vi "Dashboard Main.vi"() -> ()   [LabVIEW 2012]
uses:
  <vilib>/event_ctls.llb/eventvkey.ctl
  <vilib>/Utility/miscctls.llb/LVPointTypeDef.ctl
  <vilib>/Utility/config.llb/Read Key (String).vi
  <vilib>/Utility/config.llb/Read Key (I32).vi
  <vilib>/Utility/config.llb/Write Key (String).vi
  <vilib>/Utility/config.llb/Write Key (I32).vi
  <vilib>/Utility/config.llb/NI_LVConfig.lvlib
panel:
  in  "Camera Settings":T1={"Frate Rate"=30, "Compression"=51, "Size"=1} {"Frate Rate" scale=1.0..30.0; "Size" items=["640x480", "320x240", "160x120"]}
  out "Mode":T2(ring)=enum.""
  out "Camera IP":string="0.0.0.11"
  in  "Dashboard Tab":T3(tab)
  out "GO!! GO!! GO!!":bool
  out "Driver Ready":bool
  out "Shooter Speed":T4(ring)
  out "Shooter Encoder\nDead!!":bool
  out "Shooter Good":bool
  out "Dashboard Code Verzion":string
  out "Robot Code Version":string
  out "Display Loop speed (Hz)":dbl
  out "Shooter Good":bool
  out "Shooter Speed":dbl(graph)
  out "Wheel Speed":dbl
  out "Shooter Output":dbl
  out "Shooter Speed":T4(ring)
  out "Left Encoder":dbl
  out "Right Encoder":dbl
  out "Encoder Average":dbl
  out "Left Encoder Rate":dbl
  out "Right Encoder Rate":dbl
  out "Encoder Average Rate":dbl
  out "Gyro":dbl
  out "Battery Value":dbl(slide) scale=0.0..14.0 scale format="%#_2e"
  out "Battery":sgl(graph)
  out "JS1 Z":dbl(slide) scale=-1.0..1.0 scale format="%#_2e"
  out "JS2 Z":dbl(slide) scale=-1.0..1.0 scale format="%#_2e"
  out "Joystick 1":cluster{"X":dbl, "Y":dbl}[](graph)
  out "Joystick 2":cluster{"X":dbl, "Y":dbl}[](graph)
  out "JS Buttons 1":T5
  out "JS Buttons 2":T5
  out "MotorSlide4":dbl(slide) scale=-1.0..1.0 scale format="%#_2e"
  out "MotorSlide3":dbl(slide) scale=-1.0..1.0 scale format="%#_2e"
  out "MotorSlide2":dbl(slide) scale=-1.0..1.0 scale format="%#_2e"
  in  "MotorName3":string="Front Left"
  in  "MotorName4":string="Front Right"
  in  "MotorName1":string="Rear Left"
  in  "MotorName2":string="Rear Right"
  out "MotorChart4":dbl(graph)
  out "MotorChart3":dbl(graph)
  out "MotorChart2":dbl(graph)
  out "MotorSlide1":dbl(slide) scale=-1.0..1.0 scale format="%#_2e"
  out "MotorChart1":dbl(graph)
  out "Robot IP":string="0.0.0.0"
  in  "Slider":dbl(slide) scale=0.0..100.0 scale format="%#_3g"
  in  "On/Off":bool caption="Solenoid"
  in  "Test Name":u16(ring) items=["Select the test to run...", "Example Test", "-------------------------------", "List of tests is built in robot code.", "Replace with your own automated tests."]
  in  "Test Tree":string(tree)
  in  "Motor":cluster{"Value":dbl, "Enable":bool} {"Value" scale=-1.0..1.0 scale format="%#_3g"}
  out "Progress":T6 {"Test Progress" scale=0.0..100.0}
  in  "Rev/Fwd":cluster{"Forward":bool, "Reverse":bool}
  in  "Ring":u16(ring) items=["Auto", "Fixed indoor", "Fixed outdoor 1", "Fixed outdoor 2", "Fixed fluorescent 1", "Fixed fluorescent 2", "Hold current"]
  in  "Debug Mode":bool
  in  "Listbox":i32(listbox)
  in  "Viewer":T7(tab)
  in  "Enable Processing":bool
  out "Mbps":dbl format="%#.1g"
  in  "Enable":bool=TRUE
  in  "DB Camera Config":bool
  out "Mbps":bool
  out "fps":dbl format="%#.1g"
  out "Image Error Message":string="Timeout in Camera Communications"
  out "Camera Image":T8(plugin-control)
  out "Vision Angle":dbl
  out "Buttons 1":cluster{"1":bool, "2":bool, "3":bool}
  out "Kinect 1":cluster{"X":dbl, "Y":dbl, "Z":dbl} {"X" scale=1.0..-1.0; "Y" scale=1.0..-1.0; "Z" scale=1.0..-1.0}
  out "Buttons 2":cluster{"1":bool, "2":bool, "3":bool}
  out "Kinect 2":cluster{"X":dbl, "Y":dbl, "Z":dbl} {"X" scale=1.0..-1.0; "Y" scale=1.0..-1.0; "Z" scale=1.0..-1.0}
  out "Version":string
  out "Skeleton Picture":picture
  out "Players":i8
  out "Tree":string(tree)
  # "Drive & Motors"
  # "Robot IP:"
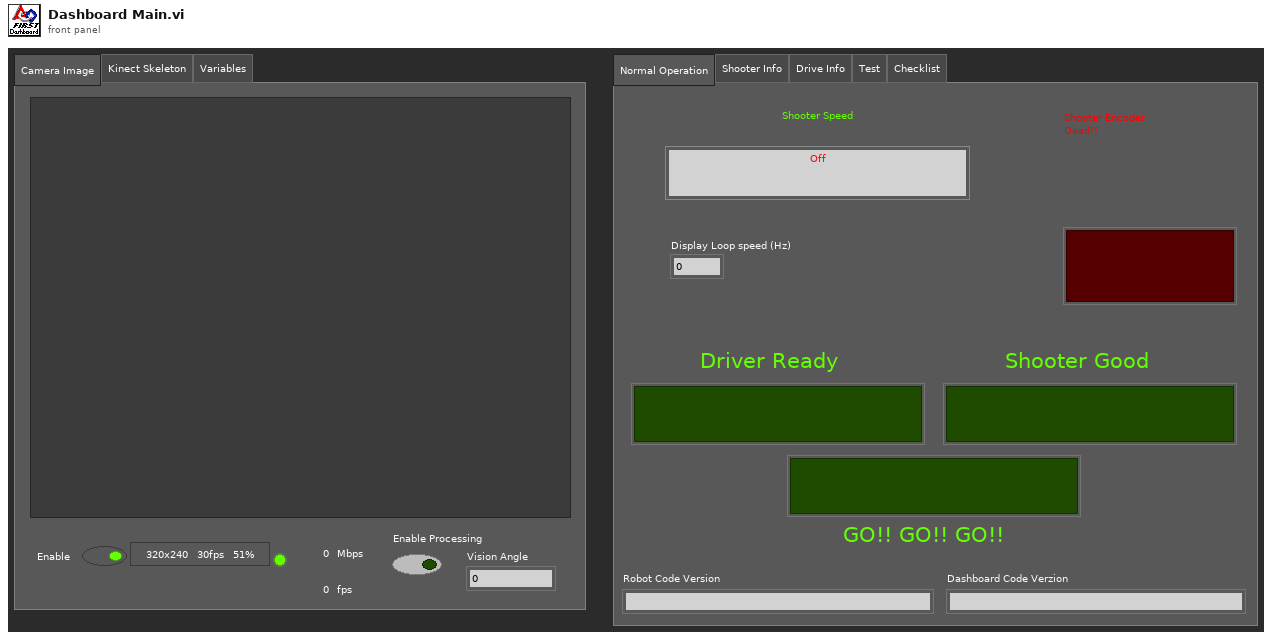
[diagram p1: front panel]
types:
  T1 = cluster{"Frate Rate":i32, "Compression":i32, "Size":u16}
  T2 = enum8{"Tele-Op Disabled", "Tele-Op Enabled", "Auto Disabled", "Auto Enabled", "Test Disabled", "Test Enabled", ""}
  T3 = enum32{"Normal Operation", "Shooter Info", "Drive Info", "Test", "Checklist"}
  T4 = enum16{"Off", "Close Pyramid 3pt", "Far Pyramid 3pt", "Feeder Shot", "UD Far 3pt Shot"}
  T5 = cluster{bool, bool, bool, bool, bool, bool, bool, bool, bool, bool, bool, bool}
  T6 = cluster{"Test Progress":u8, "Test Progress Text":string}
  T7 = enum32{"Camera Image", "Kinect Skeleton", "Variables"}
  T8 = typedef "IMAQ Image.ctl" = refnum<image>
  T9 = typedef "Image Type" = u32
  T10 = cluster{"Competition mode":bool, "Robot Link":bool, "Autonomous":bool, "Enabled":bool, "E-Stop":bool, "Simulated":bool, "TestMode":bool, "Docked Window":bool}
  T11 = cluster{"Boolean Array[0]":bool, "Boolean Array[1]":bool, "Boolean Array[2]":bool, "Boolean Array[3]":bool, "Boolean Array[4]":bool, "Boolean Array[5]":bool, "Boolean Array[6]":bool, "Boolean Array[7]":bool, "Boolean Array[8]":bool, "Boolean Array[9]":bool, "Boolean Array[10]":bool, "Boolean Array[11]":bool}
  T12 = typedef "LVPointTypeDef.ctl" = cluster{"Horizontal":i16, "Vertical":i16}
  T13 = typedef "LVRectTypeDef.ctl" = cluster{"Left":i16, "Top":i16, "Right":i16, "Bottom":i16}
  T14 = typedef "LVBoundsTypeDef.ctl" = cluster{"Width":u32, "Height":u32}
  T15 = typedef "SkeletonTrackState.ctl" = enum32{"NotTracked", "PositionOnly", "Tracked"}
  T16 = cluster{"TrackingState":u8[], "Position":cluster{"x":sgl, "y":sgl, "z":sgl}, cluster{"x":sgl, "y":sgl, "z":sgl, sgl}[], "TrackState":T15}
  T17 = cluster{cluster{"ScaledToPercentRange":dbl, "ScaledToPercentRange":dbl, "ScaledToPercentRange":dbl}, cluster{bool, bool, bool}}[]
  T18 = cluster{cluster{"ScaledToPercentRange":dbl, "ScaledToPercentRange":dbl, "ScaledToPercentRange":dbl}, cluster{bool, bool, bool}}
  T19 = cluster{"ScaledToPercentRange":dbl, "ScaledToPercentRange":dbl, "ScaledToPercentRange":dbl}
  T20 = typedef "NI_LVConfig.lvlib/Config Data RefNum.ctl" = refnum<k1>
  T21 = typedef "eventvkey.ctl" = enum16{"ASCII", "Enter", "Return", "Shift", "Ctrl", "Alt", "Cmd", "Opt", "Caps", "NumLock", "Clear", "Break", "Up", "Down", "Left", "Right", "Insert", "Delete", "Home", "End", "PageUp", "PageDown", "Escape", "Help", "Pause", "ScrollLock", "F1", "F2", "F3", "F4", "F5", "F6", "F7", "F8", "F9", "F10", "F11", "F12", "F13", "F14", "F15", "F16", "F17", "F18", "F19", "F20", "F21", "F22", "F23", "F24", "Play", "VolumeUp", "VolumeDown", "Mute", "Two Byte Char"}
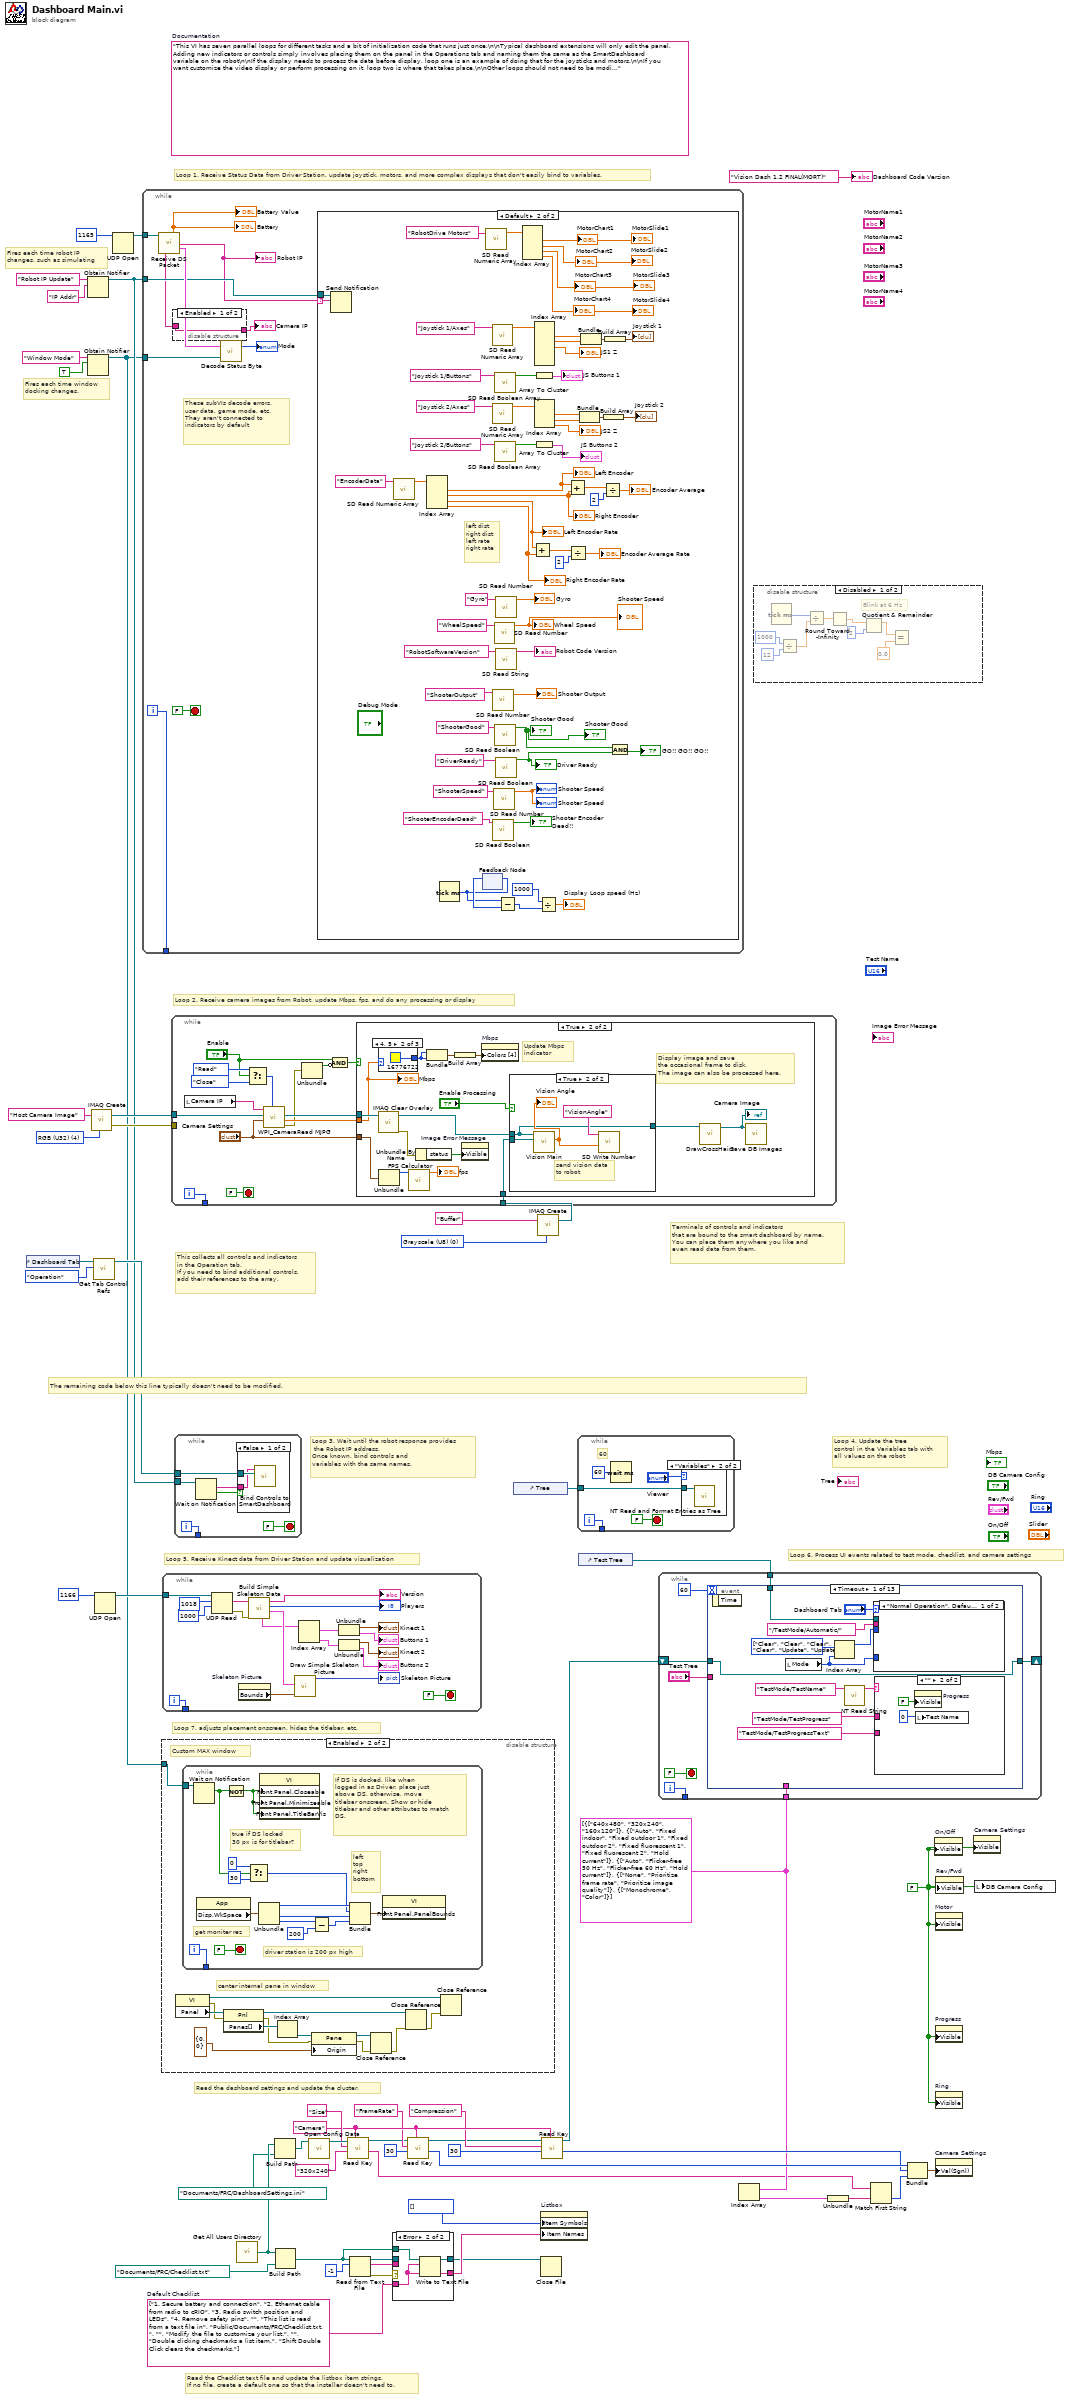
[diagram p0: block diagram]
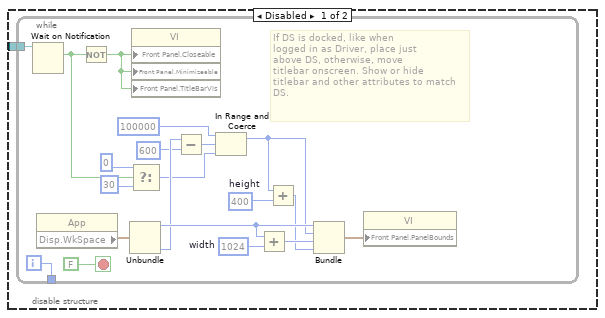
[diagram p3: hidden frame]
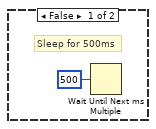
[diagram p5: hidden frame]
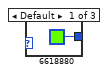
[diagram p7: hidden frame]
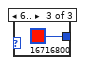
[diagram p8: hidden frame]
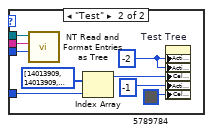
[diagram p10: hidden frame]
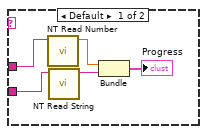
[diagram p11: hidden frame]
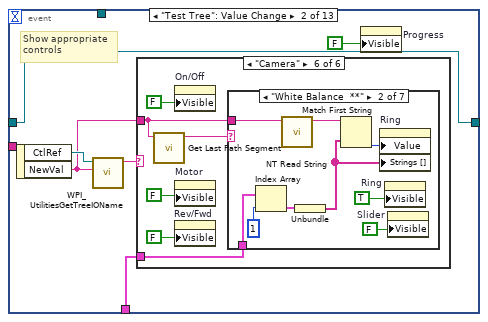
[diagram p12: hidden frame]
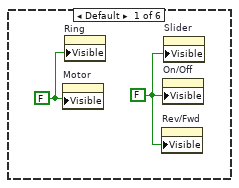
[diagram p13: hidden frame]
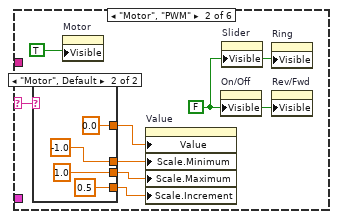
[diagram p14: hidden frame]
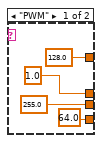
[diagram p15: hidden frame]
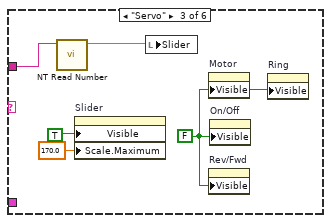
[diagram p16: hidden frame]
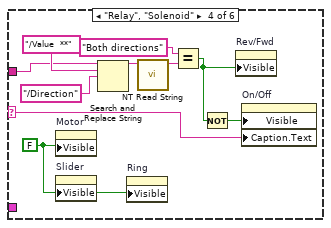
[diagram p17: hidden frame]
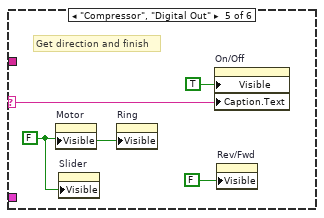
[diagram p18: hidden frame]
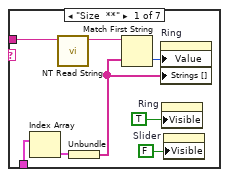
[diagram p19: hidden frame]
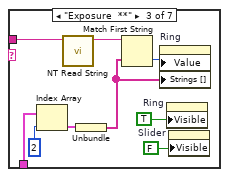
[diagram p20: hidden frame]
diagram:
  w3 = T9 0 items=["Grayscale (U8)", "Grayscale (I16)", "Grayscale (SGL)", "Complex (CSG)", "RGB (U32)", "HSL (U32)", "RGB (U64)", "Grayscale (U16)"] ("Image Type")
  w25 = "Camera"
  w17 = cluster{string[]}[] [{["640x480", "320x240", "160x120"]}, {["Auto", "Fixed indoor", "Fixed outdoor 1", "Fixed outdoor 2", "Fixed fluorescent 1", "Fixed fluorescent 2", "Hold current"]}, {["Auto", "Flicker-free 50 Hz", "Flicker-free 60 Hz", "Hold current"]}, {["None", "Prioritize frame rate", "Prioritize image quality"]}, {["Monochrome", "Color"]}]
  w33 = string[] ["1. Secure battery and connection", "2. Ethernet cable from radio to cRIO", "3. Radio switch position and LEDs", "4. Remove safety pins", "", "This list is read from a text file in", "Public/Documents/FRC/Checklist.txt.", "", "Modify the file to customize your list.", "", "Double clicking checkmarks a list item.", "Shift Double Click clears the checkmarks."]  # Default Checklist
  w31 = FALSE ("Visible")
  (unwired) "This VI has seven parallel loops for different tasks and a bit of initialization code that runs just once.\n\nTypical dashboard extensions will only edit the panel. Adding new indicators or controls simply involves placing them on the panel in the Operations tab and naming them the same as the SmartDashboard variable on the robot\n\nIf the display needs to process the data before display, loop one is an example of doing that for the joysticks and motors.\n\nIf you want customize the video display or perform processing on it, loop two is where that takes place.\n\nOther loops should not need to be modified. They are pretty standard, and document the task they perform."  # Documentation
  w54 = T9 4 items=["Grayscale (U8)", "Grayscale (I16)", "Grayscale (SGL)", "Complex (CSG)", "RGB (U32)", "HSL (U32)", "RGB (U64)"] ("Image Type")
  # "Fires each time robot IP\nchanges, such as simulating"
  # "Fires each time window\ndocking changes."
  # "Read the Checklist text file and update the listbox item strings.\nIf no file, create a default one so that the installer doesn't need to."
  # "This collects all controls and indicators\nin the Operation tab.\nIf you need to bind additional controls,\nadd their references to the array."
  # "The remaining code below this line typically doesn't need to be modified."
  # "Loop 6. Process UI events related to test mode, checklist, and camera settings"
  # "Read the dashboard settings and update the cluster."
  # "Terminals of controls and indicators\nthat are bound to the smart dashboard by name.\nYou can place them anywhere you like and\neven read data from them."
  # "Loop 4. Update the tree\ncontrol in the Variables tab with\nall values on the robot"
  # "Loop 3. Wait until the robot response provides\n the Robot IP address.\nOnce known, bind controls and\nvariables with the same names."
  # "Loop 5. Receive Kinect data from Driver Station and update visualization"
  # "Loop 7. adjusts placement onscreen, hides the titlebar, etc."
  # "Loop 1. Receive Status Data from Driver Station, update joystick, motors, and more complex displays that don't easily bind to variables."
  # "Loop 2. Receive camera images from Robot, update Mbps, fps, and do any processing or display"
  n1 = control-ref of="Dashboard Tab"() -> (w47:refnum<vi>)
  n2 = Obtain Notifier(name (unnamed)="Robot IP Update", notification data type="IP Addr" ("name (unnamed)")) -> (notifier out=w44:refnum<notifier>)  [unwired: 2 in, 2 out]
  n3 = Obtain Notifier(name (unnamed)="Window Mode", notification data type=TRUE) -> (notifier out=w37:refnum<notifier>)  [unwired: 2 in, 2 out]
  n4 = call "IMAQ Create"("Image Name"="Host Camera Image", "Image Type"=w54) -> ("New Image"=w52:T8, "error out"=w51:errorcluster)  [unwired: 2 in, 1 out]
  n5 = call <vilib>:"Get Tab Control Refs.vi"("Page Index"=enum32{"Operation", "Test"}."Operation" ("Dashboard Tab"), "TabControl in"=w47) -> ("ControlsOnPage"=w48:refnum<vi>[])  [unwired: 9 in]
  n6 = UDP Open(11:u16 1166 ("port")) -> (port=w49:refnum<k16>)  [unwired: 2 in, 4 out]
  n7 = UDP Open(11:u16 1165 ("port")) -> (port=w55:refnum<k16>)  [unwired: 2 in, 4 out]
  n8 = while {
    tunnel: w55 -> [w65]
    tunnel: w44 -> [w60]
    tunnel: w37 -> [w63]
    tunnel: [w61] -> _
    i -> [w61]
    stop <- FALSE stop-if-true
    # "These subVIs decode errors, user data, game mode, etc.\nThey aren't connected to indicators by default"
    n9 = call "Receive DS Packet.vi"("Recv Socket"=w65) -> ("Battery"=→"Battery" →"Battery Value":sgl, "Robot IP Address"=w59:string, "Status"=w66:T10, "Camera IP Address"=w57:string)  [unwired: 1 in, 10 out]
    "Robot IP" <- w59
    n10 = disable-structure shown="Enabled" {
      disable-tunnel: [w68 "10.16.76.11" ("Camera IP")] -> w58
      disable-tunnel: w57 -> [w68 _]
      frame Enabled {
      }
      frame Disabled {
      }
    }
    "Camera IP" <- w58
    n11 = call "Decode Status Byte.vi"("Window Mode Notifier"=w63, "Status"=w66) -> ("Mode"=→"Mode":T2)  [unwired: 1 out]
    n12 = case shown="Default" w59 {
      selector: w59 -> [_ w104]
      tunnel: w60 -> [_ w105]
      frame "0.0.0.0" {
        # "Robot not responding, don't poll the variables"
      }
      frame Default {
        # "left dist\nright dist\nleft rate\nright rate"
        n13 = Send Notification(notification=w104, notifier=w105) -> ()  [unwired: 1 in, 2 out]
        n14 = call <vilib>:"SD Read Numeric Array.vi"("Name"="EncoderData") -> ("Numeric Array"=w91:dbl[])  [unwired: 8 in, 2 out]
        n15 = Index Array(array=w91) -> (element #1=w90:dbl, element #2=w89:dbl, element #3=w85:dbl, element #4=w84:dbl)  [unwired: 4 in]
        "Left Encoder" <- w90
        "Right Encoder" <- w89
        "Left Encoder Rate" <- w85
        "Right Encoder Rate" <- w84
        n16 = Tick Count (ms)() -> (millisecond timer value=w73:u32)
        n17 = feedback-in #1(w73) -> ()
        n18 = feedback #1() -> (w74:u32)  [unwired: 1 in]
        n19 = call <vilib>:"SD Read Numeric Array.vi"("Name"="RobotDrive Motors") -> ("Numeric Array"=w128:dbl[])  [unwired: 8 in, 2 out]
        n20 = call <vilib>:"SD Read Numeric Array.vi"("Name"="Joystick 1/Axes") -> ("Numeric Array"=w121:dbl[])  [unwired: 8 in, 2 out]
        n21 = call <vilib>:"SD Read Numeric Array.vi"("Name"="Joystick 2/Axes") -> ("Numeric Array"=w115:dbl[])  [unwired: 8 in, 2 out]
        n22 = call <vilib>:"SD Read Number.vi"("Name"="ShooterOutput") -> ("Numeric"=→"Shooter Output":dbl)  [unwired: 8 in, 2 out]
        n23 = call <vilib>:"SD Read Boolean.vi"("Name"="ShooterEncoderDead") -> ("Boolean"=→"Shooter Encoder\nDead!!":bool)  [unwired: 8 in, 2 out]
        n24 = call <vilib>:"SD Read Number.vi"("Name"="ShooterSpeed") -> ("Numeric"=→"Shooter Speed" →"Shooter Speed":dbl)  [unwired: 8 in, 2 out]
        n25 = call <vilib>:"SD Read Number.vi"("Name"="WheelSpeed") -> ("Numeric"=→"Wheel Speed" →"Shooter Speed":dbl)  [unwired: 8 in, 2 out]
        n26 = call <vilib>:"SD Read Boolean Array.vi"("Name"="Joystick 1/Buttons") -> ("Boolean Array"=w123:bool[])  [unwired: 8 in, 2 out]
        n27 = call <vilib>:"SD Read Boolean Array.vi"("Name"="Joystick 2/Buttons") -> ("Boolean Array"=w114:bool[])  [unwired: 8 in, 2 out]
        n28 = call <vilib>:"SD Read Boolean.vi"("Name"="ShooterGood") -> ("Boolean"=w78:bool)  [unwired: 8 in, 2 out]
        "Shooter Good" <- w78
        "Shooter Good" <- w78
        n29 = call <vilib>:"SD Read Number.vi"("Name"="Gyro") -> ("Numeric"=→"Gyro":dbl)  [unwired: 8 in, 2 out]
        n30 = call <vilib>:"SD Read String.vi"("Name"="RobotSoftwareVersion") -> ("String"=→"Robot Code Version":string)  [unwired: 8 in, 2 out]
        n31 = call <vilib>:"SD Read Boolean.vi"("Name"="DriverReady") -> ("Boolean"=w77:bool)  [unwired: 8 in, 2 out]
        "Driver Ready" <- w77
        n32 = Subtract(x=w73, y=w74) -> (x-y=w72:u32)
        n33 = Index Array(array=w128) -> (element #1=→"MotorChart1" →"MotorSlide1":dbl, element #2=→"MotorSlide2" →"MotorChart2":dbl, element #3=→"MotorChart3" →"MotorSlide3":dbl, element #4=→"MotorChart4" →"MotorSlide4":dbl)  [unwired: 4 in]
        n34 = Add(x=w85, y=w84) -> (x+y=w86:dbl)
        n35 = Array To Cluster(array=w123) -> (cluster=→"JS Buttons 1":T11)
        n36 = Array To Cluster(array=w114) -> (cluster=→"JS Buttons 2":T11)
        n37 = Index Array(array=w121) -> (element #1=w118:dbl, element #2=w119:dbl, element #3=→"JS1 Z":dbl)  [unwired: 6 in, 3 out]
        n38 = Index Array(array=w115) -> (element #1=w110:dbl, element #2=w109:dbl, element #3=→"JS2 Z":dbl)  [unwired: 3 in]
        n39 = Divide(x=1000, y=w72) -> (x/y=→"Display Loop speed (Hz)":dbl)
        n40 = Add(x=w90, y=w89) -> (x+y=w100:dbl)
        n41 = Divide(x=w86, y=2) -> (x/y=→"Encoder Average Rate":dbl)
        n42 = Bundle("Numeric"=w110, "Numeric"=w109) -> (w111:cluster{"Numeric":dbl, "Numeric":dbl})  [unwired: 1 in]
        n43 = Bundle("Numeric"=w118, "Numeric"=w119) -> (w117:cluster{"Numeric":dbl, "Numeric":dbl})  [unwired: 1 in]
        n44 = Divide(x=w100, y=2) -> (x/y=→"Encoder Average":dbl)
        n45 = Build Array(w111) -> (→"Joystick 2":cluster{"Numeric":dbl, "Numeric":dbl}[])
        n46 = Build Array(w117) -> (→"Joystick 1":cluster{"Numeric":dbl, "Numeric":dbl}[])
        n47 = And(x=w78, y=w77) -> (x .and. y?=→"GO!! GO!! GO!!":bool)
      }
    }
  }
  n48 = disable-structure shown="Enabled" {
    disable-tunnel: w37 -> [w132 w165]
    frame Disabled {
      n49 = while {
        tunnel: w132 -> [w151]
        tunnel: [w149] -> _
        i -> [w149]
        stop <- FALSE stop-if-true
        w141 = 1024  # width
        w144 = 400  # height
        # "If DS is docked, like when\nlogged in as Driver, place just\nabove DS, otherwise, move\ntitlebar onscreen. Show or hide\ntitlebar and other attributes to match\nDS."
        n50 = Wait on Notification(notifier=w151) -> (notification=w136:bool)  [unwired: 3 in, 3 out]
        n51 = property class="App"() -> ("Disp.WkSpace"=w147:T13)  [unwired: 2 in, 2 out]
        n52 = Not(x=w136) -> (.not. x?=w150:bool)
        n53 = Unbundle(w147) -> ("Left"=w145:i16, "Bottom"=w142:i16)  [unwired: 2 out]
        n54 = Select(t=0, s=w136, f=30) -> (s? t:f=w135:i32)
        n55 = property class="VI"("Front Panel.Closeable"=w150, "Front Panel.Minimizeable"=w150, "Front Panel.TitleBarVis"=w150) -> ()  [unwired: 2 in, 2 out]
        n56 = Subtract(x=w142, y=600) -> (x-y=w139:i32)
        n57 = In Range and Coerce(upper limit=100000, x=w139, lower limit=w135) -> (coerced(x)=w133:i32)  [unwired: 1 out]
        n58 = Add(x=w145, y=w141) -> (x+y=w146:i32)
        n59 = Add(x=w133, y=w144) -> (x+y=w143:i32)
        n60 = Bundle("Left"=w145, w133, w146, w143) -> (w148:cluster{"Left":i16, i32, i32, i32})  [unwired: 1 out]
        n61 = property class="VI"("Front Panel.PanelBounds"=w148) -> ()  [unwired: 2 in, 2 out]
      }
    }
    frame Enabled {
      # "center internal pane in window"
      # "Custom MAX window"
      n62 = property class="VI"() -> (reference out=w158:refnum<vi>, error out=w157:errorcluster, "Panel"=w164:refnum<vi>)  [unwired: 2 in]
      n63 = while {
        tunnel: w165 -> [w179]
        tunnel: [w177] -> _
        i -> [w177]
        stop <- FALSE stop-if-true
        # "driver station is 200 px high"
        # "true if DS locked\n30 px is for titlebar?"
        # "left\ntop\nright\nbottom"
        # "get moniter rez"
        # "If DS is docked, like when\nlogged in as Driver, place just\nabove DS, otherwise, move\ntitlebar onscreen. Show or hide\ntitlebar and other attributes to match\nDS."
        n64 = Wait on Notification(notifier=w179) -> (notification=w171:bool)  [unwired: 3 in, 3 out]
        n65 = property class="App"() -> ("Disp.WkSpace"=w175:T13)  [unwired: 2 in, 2 out]
        n66 = Not(x=w171) -> (.not. x?=w178:bool)
        n67 = Select(t=0, s=w171, f=30) -> (s? t:f=w169:i32)
        n68 = Unbundle(w175) -> ("Left"=w174:i16, "Right"=w170:i16, "Bottom"=w167:i16)  [unwired: 1 out]
        n69 = property class="VI"("Front Panel.Closeable"=w178, "Front Panel.Minimizeable"=w178, "Front Panel.TitleBarVis"=w178) -> ()  [unwired: 2 in, 2 out]
        n70 = Subtract(x=w167, y=i16 200) -> (x-y=w168:i16)
        n71 = Bundle("Left"=w174, w169, "Right"=w170, w168) -> (w176:cluster{"Left":i16, i32, "Right":i16, i16})  [unwired: 1 out]
        n72 = property class="VI"("Front Panel.PanelBounds"=w176) -> ()  [unwired: 2 in, 2 out]
      }
      n73 = property class="Pnl"(reference=w164, error in=w157) -> (reference out=w159:refnum<vi>, error out=w156:errorcluster, "Panes[]"=w163:refnum<vi>[])
      n74 = Index Array(array=w163) -> (element=w162:refnum<vi>)  [unwired: 1 in]
      n75 = property class="Pane"(reference=w162, error in=w156, "Origin"=T12 {"Horizontal"=0, "Vertical"=0}) -> (reference out=w160:refnum<vi>, error out=w155:errorcluster)
      n76 = Close Reference(reference=w160, error in (no error)=w155) -> (error out=w154:errorcluster)
      n77 = Close Reference(reference=w159, error in (no error)=w154) -> (error out=w153:errorcluster)
      n78 = Close Reference(reference=w158, error in (no error)=w153) -> ()  [unwired: 1 out]
    }
  }
  n79 = while {
    tunnel: w49 -> [w197]
    tunnel: [w182] -> _
    i -> [w182]
    stop <- FALSE stop-if-true
    n80 = UDP Read(connection ID=w197, max size (548)=1018 ("bytes to read"), timeout ms (25000)=1000) -> (data out=w191:string, error out=w181:errorcluster)  [unwired: 1 in, 3 out]
    n81 = property on="Skeleton Picture" class="Pict"() -> ("Bounds"=w193:T14)  [unwired: 2 in, 2 out]
    n82 = call "Build Simple Skeleton Data.vi"("error in (no error)"=w181, "data in"=w191) -> ("Skeleton Data"=w192:T16, "NumPlayers"=→"Players":i8, "Version String"=→"Version":string, "Simple Joystick Info"=w189:T17)  [unwired: 5 in, 1 out]
    n83 = call "Draw Simple Skeleton Picture.vi"("Bounds"=w193, "Simple Skeleton"=w192) -> ("new picture out"=→"Skeleton Picture":picture)  [unwired: 9 in]
    n84 = Index Array(array=w189) -> (element #1=w188:T18, element #2=w187:T18)  [unwired: 2 in]
    n85 = Unbundle(w188) -> (→"Kinect 1":T19, →"Buttons 1":cluster{bool, bool, bool})
    n86 = Unbundle(w187) -> (→"Kinect 2":T19, →"Buttons 2":cluster{bool, bool, bool})
  }
  n87 = while {
    tunnel: w48 -> [w205]
    tunnel: w44 -> [w202]
    tunnel: [w200] -> _
    i -> [w200]
    stop <- FALSE stop-if-true
    n88 = Wait on Notification(notifier=w202) -> (notification=w201:string, timed out?=w203:bool)  [unwired: 3 in, 2 out]
    n89 = case shown="False" w203 {
      tunnel: w205 -> [w207 _]
      tunnel: w201 -> [w206 _]
      frame False {
        n90 = call <vilib>:"Bind Controls to SmartDashboard.vi"("Bound Control Refs"=w207, "Server IP Address"=w206) -> ()  [unwired: 10 in]
      }
      frame True {
      }
    }
  }
  n91 = call "Get All Users Directory.vi"() -> ("All User Path"=w30:path)
  n92 = Build Path(base path=w30, name or relative path=path "Documents/FRC/DashboardSettings.ini") -> (appended path=w29:path)
  n93 = Build Path(base path=w30, name or relative path=path "Documents/FRC/Checklist.txt") -> (appended path=w34:path)
  n94 = call <vilib>:"Open Config Data.vi"("configuration file path"=w29) -> ("refnum"=w28:T20)  [unwired: 8 in, 2 out]
  n95 = call-poly <vilib>:"Read Key.vi"("section"=w25, "default value"="320x240", "key"="Size", "refnum"=w28) -> ("value"=w15:string, "refnum out"=w10:T20)  [unwired: 2 in, 4 out]
  n96 = Read from Text File(file (use dialog)=w34, count=-1 ("timeout ms (25000)")) -> (refnum out=w12:refnum<file>, text=w35:string[], error out=w36:errorcluster)  [unwired: 2 in, 1 out]
  n97 = case shown="Error" w36 {
    tunnel: w35 -> [w209 _]
    tunnel: [w209 w211] -> w32
    tunnel: w33 -> [_ w211]
    tunnel: w34 -> [_ w212]
    tunnel: [w208 w210] -> w11
    tunnel: w12 -> [w208 _]
    frame No Error {
    }
    frame Error {
      n98 = Write to Text File(file (use dialog)=w212, text=w211) -> (refnum out=w210:refnum<file>)  [unwired: 2 in, 2 out]
    }
  }
  n99 = call-poly <vilib>:"Read Key.vi"("section"=w25, "default value"=30, "key"="FrameRate", "refnum"=w10) -> ("value"=w20:i32, "refnum out"=w9:T20)  [unwired: 1 in, 5 out]
  n100 = control-ref of="Tree"() -> (w6:refnum<vi>)
  n101 = call "IMAQ Create"("Image Name"="Buffer", "Image Type"=w3) -> ("New Image"=w2:T8)  [unwired: 3 in, 1 out]
  n102 = while {
    tunnel: w52 -> [w223]
    tunnel: w51 -> [_]
    tunnel: [w226] -> _
    tunnel: w2 -> [w213]
    i -> [w226]
    stop <- FALSE stop-if-true
    n103 = local read "Camera IP"() -> (w225:string)
    n104 = Select(t=enum16{"Read", "Reopen", "Close"}."Read" ("Operation"), s="Enable", f=enum16{"Read", "Reopen", "Close"}."Close" ("Operation")) -> (s? t:f=w218:enum16{"Read", "Reopen", "Close"})
    n105 = call <vilib>:"WPI_CameraRead MJPG.vi"("Operation"=w218, "Camera Settings"="Camera Settings", "Image"=w223, "address"=w225) -> ("error out"=w217:errorcluster, "Bandwidth (kbps)"=w221:dbl, "Image Out"=w222:T8)  [unwired: 5 in]
    n106 = Unbundle(w217) -> ("status"=w215:bool)  [unwired: 2 out]
    n107 = Compound Arithmetic op=AND("Enable", invert w215) -> (w214:bool)
    n108 = case shown="True" w214 {
      tunnel: "Camera Settings" -> [_ w235]
      tunnel: w222 -> [_ w238]
      tunnel: w221 -> [_ w237]
      tunnel: w213 -> [_ w233]
      frame False {
        # "Sleep for 500ms"
        n109 = Wait Until Next ms Multiple(millisecond multiple=u32 500) -> ()  [unwired: 1 out]
      }
      frame True {
        # "Display image and save\nthe occasional frame to disk.\nThe image can also be processed here."
        # "Update Mbps\nindicator"
        n110 = call "IMAQ Clear Overlay"("Image"=w238) -> ("error out"=w242:errorcluster, "Image Out"=w231:T8)  [unwired: 2 in, 7 out]
        n111 = case shown="4, 5" w237 {
          tunnel: [u32 6618880 ("Color Box") u32 16776722 ("Color Box") u32 16716800 ("Color Box")] -> w239
          frame Default {
          }
          frame 4, 5 {
          }
          frame 6.. {
          }
        }
        n112 = Unbundle(w235) -> ("Frate Rate"=w234:i32)  [unwired: 2 out]
        n113 = call "FPS Calculator.vi"("Average Count"=w234) -> ("fps"=→"fps":dbl)  [unwired: 10 in]
        n114 = Unbundle By Name(w242) -> ("status"=w243:bool)
        n115 = Bundle("Color Box"=w239, "Color Box"=w239) -> (w241:cluster{"Color Box":u32, "Color Box":u32})  [unwired: 1 out]
        n116 = Build Array(w241) -> (w240:cluster{"Color Box":u32, "Color Box":u32}[])
        n117 = property on="Image Error Message" class="Str"("Visible"=w243) -> ()  [unwired: 2 in, 2 out]
        n118 = property on="Mbps" class="Bool (strict)"("Colors [4]"=w240) -> ()  [unwired: 2 in, 2 out]
        n119 = case shown="True" "Enable Processing" {
          tunnel: w233 -> [_ w248]
          tunnel: w231 -> [w244 w245]
          tunnel: [w244 w245] -> w230
          frame False {
          }
          frame True {
            # "send vision data\nto robot"
            n120 = call "Vision Main.vi"("Frame Buffer"=w248, "Camera Image"=w245) -> ("Chosen Target Angle"=w246:dbl)  [unwired: 8 in, 1 out]
            "Vision Angle" <- w246
            n121 = call <vilib>:"SD Write Number.vi"("Numeric"=w246, "Name"="VisionAngle") -> ()  [unwired: 8 in, 2 out]
          }
        }
        n122 = call "DrawCrossHairs.vi"("Image In"=w230) -> ("Image Out"=w232:T8)  [unwired: 10 in]
        "Camera Image" <- w232
        n123 = call "Save DB Images.vi"("Image"=w232) -> ()  [unwired: 2 in, 1 out]
        "Mbps" <- w237
      }
    }
  }
  n124 = property on="Listbox" class="LstBox (strict)"("Item Symbols"=i32[] [], "Item Names"=w32) -> ()  [unwired: 2 in, 2 out]
  n125 = Close File(refnum=w11) -> ()  [unwired: 1 in, 2 out]
  n126 = call-poly <vilib>:"Read Key.vi"("section"=w25, "default value"=30, "key"="Compression", "refnum"=w9) -> ("value"=w19:i32, "refnum out"=w7:T20)  [unwired: 1 in, 5 out]
  n127 = while {
    tunnel: [w253] -> _
    tunnel: w6 -> [w252]
    i -> [w253]
    stop <- FALSE stop-if-true
    # "60"
    n128 = Wait (ms)(milliseconds to wait=u32 60) -> ()  [unwired: 1 out]
    n129 = case shown="\"Variables\"" "Viewer" {
      tunnel: w252 -> [_ w257]
      frame Default {
      }
      frame "Variables" {
        n130 = call <vilib>:"NT Read and Format Entries as Tree.vi"("Tree Refnum"=w257) -> ()  [unwired: 9 in, 2 out]
      }
    }
  }
  n131 = control-ref of="Test Tree"() -> (w5:refnum<vi>)
  n132 = while {
    tunnel: w17 -> [w262]
    shift-right: [w261] -> _
    shift-left: w7 -> [w260]
    tunnel: [w259] -> _
    tunnel: w5 -> [w258]
    i -> [w259]
    stop <- FALSE stop-if-true
    n133 = event shown="[0] Timeout" {
      selector: _ -> [_ _ _ _ _ _ _ _ _ _ _ _ _]
      dyn-events: _ -> [_ _ _ _ _ _ _ _ _ _ _ _ _]
      timeout: u32 60 ("milliseconds to wait") -> [_ _ _ _ _ _ _ _ _ _ _ _ _]
      tunnel: w258 -> [w272 _ _ _ _ _ _ _ _ _ _ _ _]
      tunnel: "Test Tree" -> [_ _ _ _ _ _ _ _ w466 w474 w476 w480 w488]
      tunnel: w262 -> [_ w294 _ _ _ _ w430 w460 _ _ _ _ _]
      tunnel: [w266 w293 _ w396 w404 w416 w429 w453 w465 w472 w475 w479 w487] -> w261
      tunnel: w260 -> [w266 w293 _ w396 w404 w416 w428 w453 w465 w472 w475 w479 w487]
      event Timeout {
        w271 = enum16{"Update", "Clear"}[] [enum."Clear", enum."Clear", enum."Clear", enum."Clear", enum."Update", enum."Update", enum."Clear"] items=["Update", "Clear"]
        n134 = event-data() -> ()  [unwired: 1 in, 1 out]
        n135 = local read "Mode"() -> (w269:T2)
        n136 = Index Array(array=w271, index=w269) -> (element=w270:enum16{"Update", "Clear"})
        n137 = call <vilib>:"NT Read String.vi"("Name"="TestMode/TestName") -> ("String"=w275:string)  [unwired: 9 in, 1 out]
        n138 = case shown="\"Normal Operation\", Default" "Dashboard Tab" {
          tunnel: w272 -> [_ w285]
          tunnel: "/TestMode/Automatic/" ("Name Pattern") -> [_ w284]
          tunnel: w270 -> [_ w283]
          tunnel: w269 -> [_ w281]
          frame "Normal Operation", Default {
          }
          frame "Test" {
            w280 = -2 ("Active Item:Row Number")
            n139 = call <vilib>:"NT Read and Format Entries as Tree.vi"("Operation"=w283, "Name Pattern"=w284, "Tree Refnum"=w285) -> ()  [unwired: 7 in, 2 out]
            n140 = Index Array(array=u32[] [14013909, 14013909, 14013909, 14013909, 14013909, 16777215, 14013909], index=w281) -> (element=w279:u32)
            n141 = property on="Test Tree" class="Tree (strict)"("Active Item Row Number"=w280, "ActiveColNum"=w280, "CellBG"=w279, "Active Item Row Number"=-1 ("Active Item:Row Number"), "CellBG"=u32 5789784 ("Color Box")) -> ()  [unwired: 2 in, 2 out]
          }
        }
        n142 = case shown="\"\"" w275 {
          tunnel: "TestMode/TestProgress" ("Name") -> [w287 _]
          tunnel: "TestMode/TestProgressText" ("Name") -> [w286 _]
          frame Default {
            n143 = call <vilib>:"NT Read Number.vi"("Name"=w287) -> ("Numeric"=w288:dbl)  [unwired: 9 in, 1 out]
            n144 = call <vilib>:"NT Read String.vi"("Name"=w286) -> ("String"=w289:string)  [unwired: 9 in, 1 out]
            n145 = Bundle("Numeric"=w288, "String"=w289) -> (→"Progress":cluster{"Numeric":dbl, "String":string})  [unwired: 1 in]
          }
          frame "" {
            n146 = property on="Progress" class="Clust (strict)"("Visible"=FALSE) -> ()  [unwired: 2 in, 2 out]
            n147 = local write "Test Name"(u16 0) -> ()
          }
        }
      }
      event "Test Tree": Value Change {
        # "Show appropriate\ncontrols"
        n148 = event-data() -> ("CtlRef"=w297:refnum<vi>, "NewVal"=w295:string)  [unwired: 1 in]
        n149 = call <vilib>:"WPI_UtilitiesGetTreeIOName.vi"("NewVal"=w295, "TreeControl in"=w297) -> ("I/O Name"=w298:string)  [unwired: 9 in]
        n150 = case shown="\"Camera\"" w298 {
          selector: w298 -> [_ w305 _ w323 w332 _]
          tunnel: w295 -> [_ _ w320 w322 _ w339]
          tunnel: w294 -> [_ _ _ _ _ w338]
          frame Default {
            w300 = FALSE ("Visible")
            w299 = FALSE ("Visible")
            n151 = property on="Motor" class="Clust (strict)"("Visible"=w299) -> ()  [unwired: 2 in, 2 out]
            n152 = property on="Ring" class="Ring (strict)"("Visible"=w299) -> ()  [unwired: 2 in, 2 out]
            n153 = property on="Rev/Fwd" class="Clust (strict)"("Visible"=w300) -> ()  [unwired: 2 in, 2 out]
            n154 = property on="On/Off" class="Bool (strict)"("Visible"=w300) -> ()  [unwired: 2 in, 2 out]
            n155 = property on="Slider" class="Slide (strict)"("Visible"=w300) -> ()  [unwired: 2 in, 2 out]
          }
          frame "Motor", "PWM" {
            w306 = FALSE ("Visible")
            n156 = case shown="\"Motor\", Default" w305 {
              tunnel: [1.0 ("Value") -1.0 ("Value")] -> w304
              tunnel: [255.0 ("Value") 1.0 ("Value")] -> w303
              tunnel: [128.0 ("Value") 0.0 ("Value")] -> w302
              tunnel: [64.0 ("Value") 0.5 ("Value")] -> w301
              frame "PWM" {
              }
              frame "Motor", Default {
              }
            }
            n157 = property on="Motor" class="Clust (strict)"("Visible"=TRUE) -> ()  [unwired: 2 in, 2 out]
            n158 = property on="Value" class="Slide (strict)"("Value"=w302, "Scale.Minimum"=w304, "Scale.Maximum"=w303, "Scale.Increment"=w301) -> ()  [unwired: 2 in, 2 out]
            n159 = property on="On/Off" class="Bool (strict)"("Visible"=w306) -> ()  [unwired: 2 in, 2 out]
            n160 = property on="Slider" class="Slide (strict)"("Visible"=w306) -> ()  [unwired: 2 in, 2 out]
            n161 = property on="Ring" class="Ring (strict)"("Visible"=w306) -> ()  [unwired: 2 in, 2 out]
            n162 = property on="Rev/Fwd" class="Clust (strict)"("Visible"=w306) -> ()  [unwired: 2 in, 2 out]
          }
          frame "Servo" {
            w318 = FALSE ("Visible")
            n163 = call <vilib>:"NT Read Number.vi"("Name"=w320) -> ("Numeric"=w319:dbl)  [unwired: 9 in, 1 out]
            n164 = property on="Slider" class="Slide (strict)"("Visible"=TRUE, "Scale.Maximum"=170.0 ("Scale.Range:Maximum")) -> ()  [unwired: 2 in, 2 out]
            n165 = local write "Slider"(w319) -> ()
            n166 = property on="Motor" class="Clust (strict)"("Visible"=w318) -> ()  [unwired: 2 in, 2 out]
            n167 = property on="Rev/Fwd" class="Clust (strict)"("Visible"=w318) -> ()  [unwired: 2 in, 2 out]
            n168 = property on="On/Off" class="Bool (strict)"("Visible"=w318) -> ()  [unwired: 2 in, 2 out]
            n169 = property on="Ring" class="Ring (strict)"("Visible"=w318) -> ()  [unwired: 2 in, 2 out]
          }
          frame "Relay", "Solenoid" {
            w321 = FALSE ("Visible")
            n170 = property on="Motor" class="Clust (strict)"("Visible"=w321) -> ()  [unwired: 2 in, 2 out]
            n171 = property on="Slider" class="Slide (strict)"("Visible"=w321) -> ()  [unwired: 2 in, 2 out]
            n172 = Search and Replace String(input string=w322, search string="/Value  **", replace string="/Direction") -> (result string=w328:string)  [unwired: 5 in, 3 out]
            n173 = property on="Ring" class="Ring (strict)"("Visible"=w321) -> ()  [unwired: 2 in, 2 out]
            n174 = call <vilib>:"NT Read String.vi"("Name"=w328) -> ("String"=w326:string)  [unwired: 9 in, 1 out]
            n175 = Equal?(x="Both directions", y=w326) -> (x = y?=w324:bool)
            n176 = Not(x=w324) -> (.not. x?=w325:bool)
            n177 = property on="Rev/Fwd" class="Clust (strict)"("Visible"=w324) -> ()  [unwired: 2 in, 2 out]
            n178 = property on="On/Off" class="Bool (strict)"("Visible"=w325, "Caption.Text"=w323) -> ()  [unwired: 2 in, 2 out]
          }
          frame "Compressor", "Digital Out" {
            w331 = FALSE ("Visible")
            # "Get direction and finish"
            n179 = property on="Motor" class="Clust (strict)"("Visible"=w331) -> ()  [unwired: 2 in, 2 out]
            n180 = property on="Slider" class="Slide (strict)"("Visible"=w331) -> ()  [unwired: 2 in, 2 out]
            n181 = property on="Ring" class="Ring (strict)"("Visible"=w331) -> ()  [unwired: 2 in, 2 out]
            n182 = property on="On/Off" class="Bool (strict)"("Visible"=TRUE, "Caption.Text"=w332) -> ()  [unwired: 2 in, 2 out]
            n183 = property on="Rev/Fwd" class="Clust (strict)"("Visible"=FALSE) -> ()  [unwired: 2 in, 2 out]
          }
          frame "Camera" {
            n184 = call <vilib>:"Get Last Path Segment.vi"("String in"=w339) -> ("String out"=w340:string)  [unwired: 10 in]
            n185 = property on="On/Off" class="Bool (strict)"("Visible"=FALSE) -> ()  [unwired: 2 in, 2 out]
            n186 = property on="Motor" class="Clust (strict)"("Visible"=FALSE) -> ()  [unwired: 2 in, 2 out]
            n187 = property on="Rev/Fwd" class="Clust (strict)"("Visible"=FALSE) -> ()  [unwired: 2 in, 2 out]
            n188 = case shown="\"White Balance  **\"" w340 {
              tunnel: w339 -> [w346 w355 w364 w373 w382 _ w388]
              tunnel: w338 -> [w344 w352 w361 w370 w379 _ _]
              frame "Size  **" {
                n189 = Index Array(array=w344) -> (element=w343:cluster{string[]})  [unwired: 1 in]
                n190 = call <vilib>:"NT Read String.vi"("Name"=w346) -> ("String"=w345:string)  [unwired: 9 in, 1 out]
                n191 = Unbundle(w343) -> (w341:string[])
                n192 = Match First String(2:w341, 3:w345) -> (0:w342:i32)  [unwired: 1 out]
                n193 = property on="Ring" class="Ring (strict)"("Value"=w342, "Strings []"=w341) -> ()  [unwired: 2 in, 2 out]
                n194 = property on="Ring" class="Ring (strict)"("Visible"=TRUE) -> ()  [unwired: 2 in, 2 out]
                n195 = property on="Slider" class="Slide (strict)"("Visible"=FALSE) -> ()  [unwired: 2 in, 2 out]
              }
              frame "White Balance  **" {
                n196 = Index Array(array=w352, index=1) -> (element=w353:cluster{string[]})
                n197 = call <vilib>:"NT Read String.vi"("Name"=w355) -> ("String"=w354:string)  [unwired: 9 in, 1 out]
                n198 = Unbundle(w353) -> (w350:string[])
                n199 = Match First String(2:w350, 3:w354) -> (0:w349:i32)  [unwired: 1 out]
                n200 = property on="Ring" class="Ring (strict)"("Value"=w349, "Strings []"=w350) -> ()  [unwired: 2 in, 2 out]
                n201 = property on="Ring" class="Ring (strict)"("Visible"=TRUE) -> ()  [unwired: 2 in, 2 out]
                n202 = property on="Slider" class="Slide (strict)"("Visible"=FALSE) -> ()  [unwired: 2 in, 2 out]
              }
              frame "Exposure  **" {
                n203 = Index Array(array=w361, index=2) -> (element=w362:cluster{string[]})
                n204 = call <vilib>:"NT Read String.vi"("Name"=w364) -> ("String"=w363:string)  [unwired: 9 in, 1 out]
                n205 = Unbundle(w362) -> (w358:string[])
                n206 = Match First String(2:w358, 3:w363) -> (0:w359:i32)  [unwired: 1 out]
                n207 = property on="Ring" class="Ring (strict)"("Value"=w359, "Strings []"=w358) -> ()  [unwired: 2 in, 2 out]
                n208 = property on="Ring" class="Ring (strict)"("Visible"=TRUE) -> ()  [unwired: 2 in, 2 out]
                n209 = property on="Slider" class="Slide (strict)"("Visible"=FALSE) -> ()  [unwired: 2 in, 2 out]
              }
              frame "Exposure Priority  **" {
                n210 = Index Array(array=w370, index=3) -> (element=w371:cluster{string[]})
                n211 = call <vilib>:"NT Read String.vi"("Name"=w373) -> ("String"=w372:string)  [unwired: 9 in, 1 out]
                n212 = Unbundle(w371) -> (w367:string[])
                n213 = Match First String(2:w367, 3:w372) -> (0:w368:i32)  [unwired: 1 out]
                n214 = property on="Ring" class="Ring (strict)"("Value"=w368, "Strings []"=w367) -> ()  [unwired: 2 in, 2 out]
                n215 = property on="Ring" class="Ring (strict)"("Visible"=TRUE) -> ()  [unwired: 2 in, 2 out]
                n216 = property on="Slider" class="Slide (strict)"("Visible"=FALSE) -> ()  [unwired: 2 in, 2 out]
              }
              frame "Color Enable  **" {
                n217 = Index Array(array=w379, index=4) -> (element=w380:cluster{string[]})
                n218 = call <vilib>:"NT Read String.vi"("Name"=w382) -> ("String"=w381:string)  [unwired: 9 in, 1 out]
                n219 = Unbundle(w380) -> (w376:string[])
                n220 = Match First String(2:w376, 3:w381) -> (0:w377:i32)  [unwired: 1 out]
                n221 = property on="Ring" class="Ring (strict)"("Value"=w377, "Strings []"=w376) -> ()  [unwired: 2 in, 2 out]
                n222 = property on="Ring" class="Ring (strict)"("Visible"=TRUE) -> ()  [unwired: 2 in, 2 out]
                n223 = property on="Slider" class="Slide (strict)"("Visible"=FALSE) -> ()  [unwired: 2 in, 2 out]
              }
              frame Default {
                n224 = property on="Ring" class="Ring (strict)"("Visible"=FALSE) -> ()  [unwired: 2 in, 2 out]
                n225 = property on="Slider" class="Slide (strict)"("Visible"=FALSE) -> ()  [unwired: 2 in, 2 out]
              }
              frame "Brightness  **", "Color Level  **", "Compression  **", "FPS  **", "Sharpness  **" {
                n226 = call <vilib>:"NT Read Number.vi"("Name"=w388) -> ("Numeric"=w387:dbl)  [unwired: 9 in, 1 out]
                n227 = local write "Slider"(w387) -> ()
                n228 = property on="Slider" class="Slide (strict)"("Visible"=TRUE, "Scale.Maximum"=100.0 ("Scale.Range:Maximum")) -> ()  [unwired: 2 in, 2 out]
                n229 = property on="Ring" class="Ring (strict)"("Visible"=FALSE) -> ()  [unwired: 2 in, 2 out]
              }
            }
          }
        }
        n230 = property on="Progress" class="Clust (strict)"("Visible"=FALSE) -> ()  [unwired: 2 in, 2 out]
      }
      event "Test Name": Mouse Enter {
        # "Populate the ring with the list of tests"
        n231 = event-data() -> ()  [unwired: 1 in, 1 out]
        n232 = call <vilib>:"NT Read String Array.vi"("Name"="TestMode/TestList") -> ("String Array"=w395:string[])  [unwired: 9 in, 1 out]
        n233 = Build Array (concatenate)("Select the test to run...", w395) -> (w394:string[])
        n234 = property on="Test Name" class="Ring (strict)"("Strings []"=w394) -> ()  [unwired: 2 in, 2 out]
      }
      event "Test Name": Value Change {
        w397 = FALSE ("Visible")
        # "Tell the robot the test name to run"
        n235 = event-data() -> ("NewVal"=w401:u16)  [unwired: 1 in]
        n236 = property on="Test Name" class="Ring (strict)"() -> ("Strings []"=w402:string[])  [unwired: 2 in, 2 out]
        n237 = local write "Progress"(T6 {"Test Progress"=0, "Test Progress Text"=""} ("Progress")) -> ()
        n238 = Index Array(array=w402, index=w401) -> (element=w400:string)
        n239 = call <vilib>:"NT Write String.vi"("String"=w400, "Name"="TestMode/TestName") -> ()  [unwired: 9 in, 1 out]
        n240 = property on="Progress" class="Clust (strict)"("Visible"=TRUE) -> ()  [unwired: 2 in, 2 out]
        n241 = property on="Motor" class="Clust (strict)"("Visible"=w397) -> ()  [unwired: 2 in, 2 out]
        n242 = property on="Slider" class="Slide (strict)"("Visible"=w397) -> ()  [unwired: 2 in, 2 out]
        n243 = property on="On/Off" class="Bool (strict)"("Visible"=w397) -> ()  [unwired: 2 in, 2 out]
        n244 = property on="Rev/Fwd" class="Clust (strict)"("Visible"=w397) -> ()  [unwired: 2 in, 2 out]
        n245 = property on="Ring" class="Ring (strict)"("Visible"=w397) -> ()  [unwired: 2 in, 2 out]
      }
      event "Listbox": Double Click {
        n246 = event-data() -> ("PlatMods.Shift"=w405:bool, "Row"=w407:i32)  [unwired: 1 in]
        n247 = case shown="False" w405 {
          tunnel: w407 -> [w411 _]
          tunnel: 1 -> [w410 _]
          frame False {
            n248 = property on="Listbox" class="LstBox (strict)"() -> ("Item Symbols"=w409:i32[])  [unwired: 2 in, 2 out]
            n249 = Replace Array Subset(array=w409, new element=w410, index=w411) -> (w408:i32[])
            n250 = property on="Listbox" class="LstBox (strict)"("Item Symbols"=w408) -> ()  [unwired: 2 in, 2 out]
          }
          frame True {
            w412 = 0 ("Top Row")
            n251 = property on="Listbox" class="LstBox (strict)"() -> ("Number of Rows"=w414:u32)  [unwired: 2 in, 2 out]
            n252 = Initialize Array(0, w414) -> (w413:i32[])
            n253 = property on="Listbox" class="LstBox (strict)"("Top Row"=w412, "Value"=w412, "Item Symbols"=w413) -> ()  [unwired: 2 in, 2 out]
          }
        }
      }
      event "Listbox": Key Down {
        n254 = event-data() -> ("VKey"=w418:T21)  [unwired: 1 in]
        n255 = case shown="\"Left\", \"Right\"" w418 {
          selector: w418 -> [w423 _]
          tunnel: eventvkey."Left" ("VKey") -> [w421 _]
          frame "Left", "Right" {
            n256 = Equal?(x=w421, y=w423) -> (x = y?=w422:bool)
            n257 = Select(t=0, s=w422, f=1) -> (s? t:f=w424:i32)
            n258 = property on="Listbox" class="LstBox (strict)"() -> ("Item Symbols"=w427:i32[])  [unwired: 2 in, 2 out]
            n259 = Replace Array Subset(array=w427, new element=w424, index="Listbox") -> (w426:i32[])
            n260 = property on="Listbox" class="LstBox (strict)"("Item Symbols"=w426) -> ()  [unwired: 2 in, 2 out]
          }
          frame Default {
          }
        }
      }
      event "DB Camera Config": Value Change {
        n261 = event-data() -> ("NewVal"=w431:bool)  [unwired: 1 in]
        n262 = case shown="False" w431 {
          tunnel: w430 -> [w440 _]
          tunnel: [w433 w451] -> w429
          tunnel: w428 -> [w432 w451]
          frame False {
            w447 = "Camera"
            w450 = FALSE ("Visible")
            n263 = local read "Camera Settings"() -> (w439:T1)
            n264 = Index Array(array=w440) -> (element=w443:cluster{string[]})  [unwired: 1 in]
            n265 = Unbundle(w439) -> ("Frate Rate"=w438:i32, "Compression"=w437:i32, "Size"=w441:u16)
            n266 = Unbundle(w443) -> (w442:string[])
            n267 = Index Array(array=w442, index=w441) -> (element=w436:string)
            n268 = call-poly <vilib>:"Write Key.vi"("section"=w447, "value"=w436, "key"="Size", "refnum"=w432) -> ("refnum out"=w449:T20)  [unwired: 2 in, 5 out]
            n269 = call-poly <vilib>:"Write Key.vi"("section"=w447, "value"=w438, "key"="FrameRate", "refnum"=w449) -> ("refnum out"=w448:T20)  [unwired: 1 in, 6 out]
            n270 = property on="Camera Settings" class="Clust (strict)"("Visible"=w450) -> ()  [unwired: 2 in, 2 out]
            n271 = local write "DB Camera Config"(w450) -> ()
            n272 = call-poly <vilib>:"Write Key.vi"("section"=w447, "value"=w437, "key"="Compression", "refnum"=w448) -> ("refnum out"=w434:T20)  [unwired: 1 in, 6 out]
            n273 = call <vilib>:"Close Config Data.vi"("refnum"=w434) -> ("file path"=w435:path)  [unwired: 2 in, 8 out]
            n274 = call <vilib>:"Open Config Data.vi"("configuration file path"=w435) -> ("refnum"=w433:T20)  [unwired: 8 in, 2 out]
          }
          frame True {
            n275 = property on="Camera Settings" class="Clust (strict)"("Visible"=TRUE) -> ()  [unwired: 2 in, 2 out]
          }
        }
      }
      event "Camera Settings": Value Change {
        n276 = event-data() -> ("NewVal"=w464:T1)  [unwired: 1 in]
        n277 = Index Array(array=w460) -> (element=w459:cluster{string[]})  [unwired: 1 in]
        n278 = Unbundle(w464) -> ("Frate Rate"=w455:i32, "Compression"=w454:i32, "Size"=w457:u16)
        n279 = Unbundle(w459) -> (w458:string[])
        n280 = Index Array(array=w458, index=w457) -> (element=w456:string)
        n281 = Format Into String(format string="%s   %dfps   %d%%", w456, w455, w454) -> (resulting string=w461:string)  [unwired: 2 in, 1 out]
        n282 = Build Array(w461) -> (w462:string[])
        n283 = property on="DB Camera Config" class="Bool (strict)"("Strings [4]"=w462) -> ()  [unwired: 2 in, 2 out]
      }
      event "Motor.Enable": Value Change {
        n284 = event-data() -> ("NewVal"=w470:bool)  [unwired: 1 in]
        n285 = Unbundle("Motor") -> ("Value"=w469:dbl)  [unwired: 1 out]
        n286 = Select(t=w469, s=w470, f=0.0) -> (s? t:f=w467:dbl)
        n287 = call <vilib>:"NT Write Number.vi"("Numeric"=w467, "Name"=w466) -> ()  [unwired: 9 in, 1 out]
      }
      event "Slider": Value Change {
        n288 = event-data() -> ("NewVal"=w473:dbl)  [unwired: 1 in]
        n289 = call <vilib>:"NT Write Number.vi"("Numeric"=w473, "Name"=w474) -> ()  [unwired: 9 in, 1 out]
      }
      event "On/Off": Value Change {
        n290 = event-data() -> ("NewVal"=w478:bool)  [unwired: 1 in]
        n291 = Boolean To (0,1)(Boolean=w478) -> (0, 1=w477:i16)
        n292 = call <vilib>:"NT Write Number.vi"("Numeric"=w477, "Name"=w476) -> ()  [unwired: 9 in, 1 out]
      }
      event "Rev/Fwd": Value Change {
        n293 = event-data() -> ("NewVal.Forward"=w486:bool, "NewVal.Reverse"=w485:bool)  [unwired: 1 in]
        n294 = Boolean To (0,1)(Boolean=w486) -> (0, 1=w482:i16)
        n295 = Boolean To (0,1)(Boolean=w485) -> (0, 1=w484:i16)
        n296 = Negate(x=w484) -> (-x=w483:i16)
        n297 = Add(x=w482, y=w483) -> (x+y=w481:i16)
        n298 = call <vilib>:"NT Write Number.vi"("Numeric"=w481, "Name"=w480) -> ()  [unwired: 9 in, 1 out]
      }
      event "Ring": Value Change {
        n299 = event-data() -> ("NewVal"=w490:u16)  [unwired: 1 in]
        n300 = property on="Ring" class="Ring (strict)"() -> ("Strings []"=w491:string[])  [unwired: 2 in, 2 out]
        n301 = Index Array(array=w491, index=w490) -> (element=w489:string)
        n302 = call <vilib>:"NT Write String.vi"("String"=w489, "Name"=w488) -> ()  [unwired: 9 in, 1 out]
      }
    }
  }
  n303 = Index Array(array=w17) -> (element=w18:cluster{string[]})  [unwired: 1 in]
  n304 = disable-structure shown="Disabled" {
    frame Disabled {
      # "Blink at 6 Hz"
      n305 = Tick Count (ms)() -> (millisecond timer value=w492:u32)
      n306 = Divide(x=1000, y=12) -> (x/y=w495:dbl)
      n307 = Divide(x=w492, y=w495) -> (x/y=w497:dbl)
      n308 = Round Toward -Infinity(1:w497) -> (0:w498:dbl)
      n309 = Quotient & Remainder(x=w498, y=2) -> (x-y*floor(x/y)=w499:dbl)  [unwired: 1 out]
      n310 = Equal?(x=w499, y=0.0) -> (x = y?=w501:bool)
    }
    frame Enabled {
    }
  }
  n311 = Unbundle(w18) -> (w16:string[])
  n312 = Match First String(2:w16, 3:w15) -> (0:w14:i32)  [unwired: 1 out]
  n313 = Bundle("value"=w20, "value"=w19, "index"=w14) -> (w8:cluster{"value":i32, "value":i32, "index":i32})  [unwired: 1 out]
  n314 = property on="On/Off" class="Bool (strict)"("Visible"=w31) -> ()  [unwired: 2 in, 2 out]
  n315 = property on="Motor" class="Clust (strict)"("Visible"=w31) -> ()  [unwired: 2 in, 2 out]
  n316 = property on="Progress" class="Clust (strict)"("Visible"=w31) -> ()  [unwired: 2 in, 2 out]
  n317 = property on="Ring" class="Ring (strict)"("Visible"=w31) -> ()  [unwired: 2 in, 2 out]
  n318 = property on="Camera Settings" class="Clust (strict)"("Val(Sgnl)"=w8) -> ()  [unwired: 2 in, 2 out]
  n319 = property on="Rev/Fwd" class="Clust (strict)"("Visible"=w31) -> ()  [unwired: 2 in, 2 out]
  n320 = property on="Camera Settings" class="Clust (strict)"("Visible"=w31) -> ()  [unwired: 2 in, 2 out]
  n321 = local write "DB Camera Config"(w31) -> ()
  "Dashboard Code Verzion" <- "Vision Dash 1.2 FINAL(MORT)" ("Dashboard Code Verzion")
